vi "Demo_NOK_PART_COUNT.vi"(0 "Refnum in":T1, 1 "Station":string, 3 "Shift":i32, 5 "MAX BREAKDOWN ID":i32, 7 "Product code":string, 9 "TABLE NAME":string, 11 "error in (no error)":errorcluster, 12 "REJECTION COUNT":i32) -> (4 "Refnum out":T1, 6 "REJ COUNT":i32, 15 "error out":errorcluster)   [LabVIEW 2017]
uses:
  <vilib>/addons/database/Connection.llb/Conn ObjectReference.ctl
  <vilib>/addons/database/NI_Database_API.lvlib
  <userlib>/_OpenG.lib/comparison/comparison.llb/I32 Changed__ogtk.vi
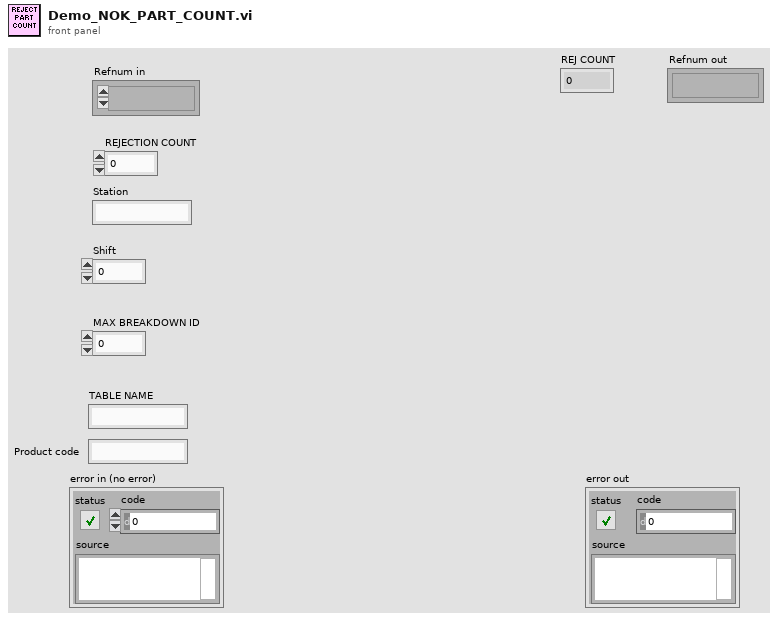
[diagram p1: front panel]
types:
  T1 = typedef "NI_Database_API.lvlib/Conn ObjectReference.ctl" = refnum<k1>
  T2 = typedef "LVDateTimeRec.ctl" = cluster{"fractional second":dbl, "second":i32, "minute":i32, "hour":i32, "day of month":i32, "month":i32, "year":i32, "day of week":i32, "day of year":i32, "DST":i32}
  T3 = cluster{i32, "Station":string, i32, "Shift":i32, "date/time string":string, "Date String":string, "Product code":string}
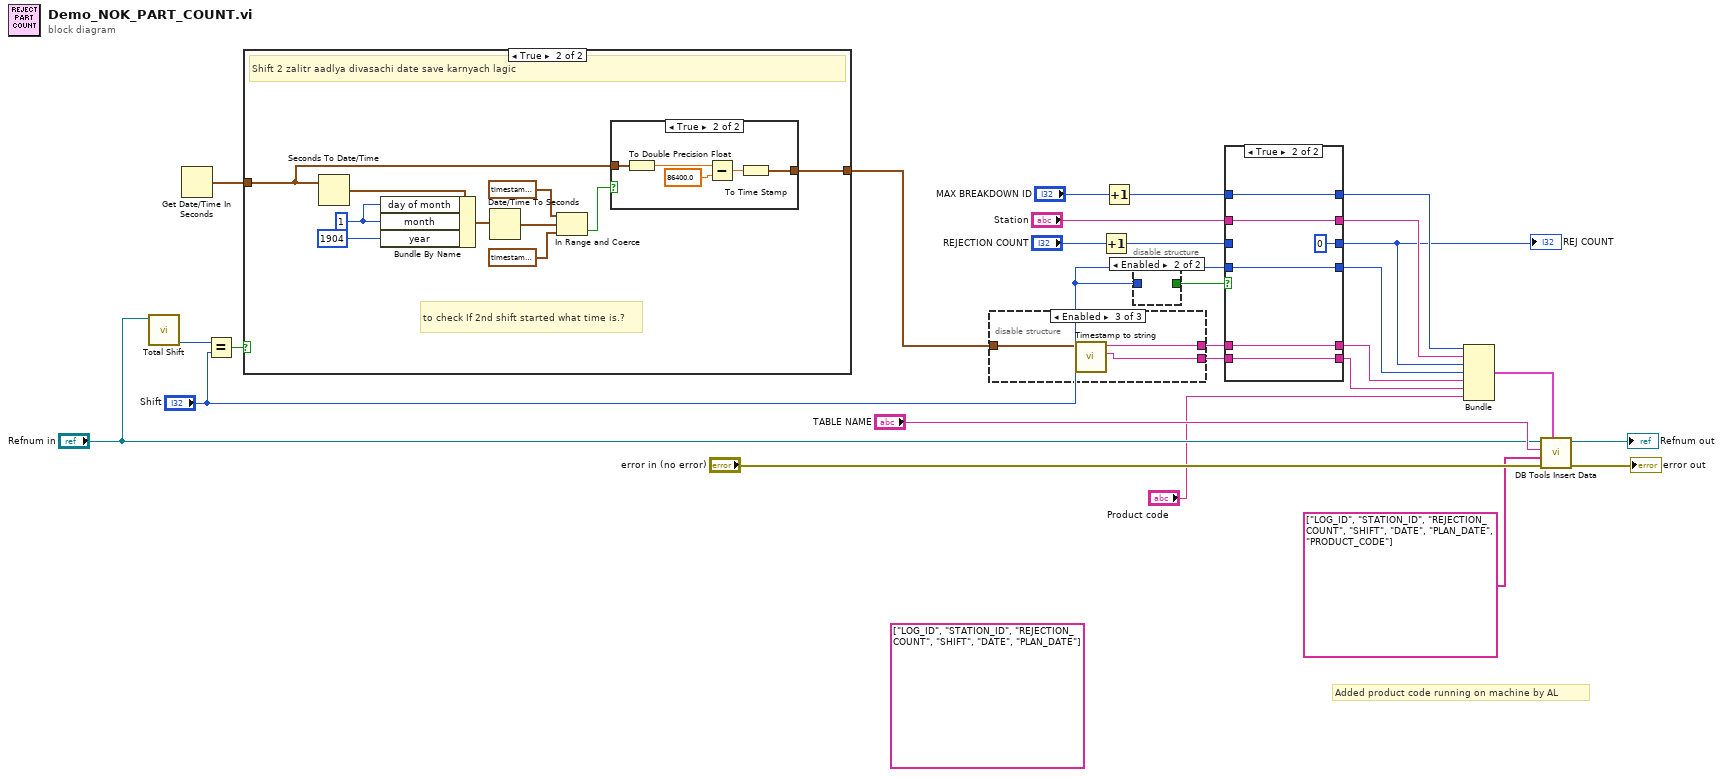
[diagram p0: block diagram]
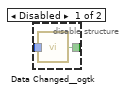
[diagram p2: hidden frame]
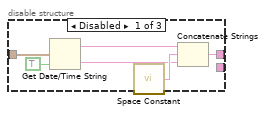
[diagram p3: hidden frame]
diagram:
  (unwired) string[] ["LOG_ID", "STATION_ID", "REJECTION_COUNT", "SHIFT", "DATE", "PLAN_DATE"] ("columns")
  # "Added product code running on machine by AL"
  n1 = call "Total Shift.vi"("connection reference"="Refnum in") -> ("Total Shifts"=w10:i32)  [unwired: 9 in, 1 out]
  n2 = Get Date/Time In Seconds() -> (seconds since 1Jan1904=w9:timestamp)
  n3 = Equal?(x=w10, y="Shift") -> (x = y?=w11:bool)
  n4 = case shown="True" w11 {
    tunnel: w9 -> [w28 w29]
    tunnel: [w28 w30] -> w8
    frame False {
    }
    frame True {
      w35 = 1 ("day of month")
      # "to check If 2nd shift started what time is.?"
      # "Shift 2 zalitr aadlya divasachi date save karnyach lagic"
      n5 = Seconds To Date/Time(time stamp (now)=w29) -> (date time rec=w36:T2)  [unwired: 1 in]
      n6 = Bundle By Name(cluster=w36, "day of month"=w35, "month"=w35, "year"=1904) -> (w38:T2)
      n7 = Date/Time To Seconds(2:w38) -> (0:w34:timestamp)  [unwired: 1 in]
      n8 = In Range and Coerce(upper limit=timestamp(5399 s since 1904-01-01), x=w34, lower limit=timestamp(-19800 s since 1904-01-01)) -> (In Range?=w31:bool)  [unwired: 1 out]
      n9 = case shown="True" w31 {
        tunnel: [w39 w41] -> w30
        tunnel: w29 -> [w39 w40]
        frame False {
        }
        frame True {
          n10 = To Double Precision Float(number=w40) -> (double precision float=w44:dbl)
          n11 = Subtract(x=w44, y=86400.0) -> (x-y=w42:dbl)
          n12 = To Time Stamp(1:w42) -> (0:w41:timestamp)
        }
      }
    }
  }
  n13 = disable-structure shown="Enabled" {
    disable-tunnel: w8 -> [w50 w51 w54]
    disable-tunnel: [w46 w51 w53] -> w5
    disable-tunnel: [_ _ w52] -> w4
    frame Disabled {
      n14 = Get Date/Time String(seconds (now)=w50, want seconds? (F)=TRUE) -> (date string=w47:string, time string=w48:string)  [unwired: 1 in]
      n15 = call <vilib>:"Space Constant.vi"() -> ("String"=w49:string)
      n16 = Concatenate Strings(w47, w49, w48) -> (w46:string)
    }
    frame Disabled {
    }
    frame Enabled {
      n17 = call "Timestamp to string.vi"("time stamp"=w54) -> ("Date String"=w52:string, "date/time string"=w53:string)  [unwired: 8 in, 1 out]
    }
  }
  n18 = Increment(x="REJECTION COUNT") -> (x+1=w15:i32)
  n19 = Increment(x="MAX BREAKDOWN ID") -> (x+1=w18:i32)
  n20 = disable-structure shown="Enabled" {
    disable-tunnel: [w56 _] -> w20
    disable-tunnel: "Shift" -> [w55 _]
    frame Disabled {
      n21 = call-poly <userlib>:"Data Changed__ogtk.vi"("I32"=w55) -> ("Changed"=w56:bool)
    }
    frame Enabled {
    }
  }
  n22 = case shown="True" w20 {
    tunnel: [w62 w68] -> w19
    tunnel: w18 -> [w62 w68]
    tunnel: [w61 w67] -> w17
    tunnel: "Station" -> [w61 w67]
    tunnel: [w60 0] -> w12
    tunnel: w15 -> [w60 _]
    tunnel: [w59 w66] -> w14
    tunnel: "Shift" -> [w59 w66]
    tunnel: [w58 w65] -> w13
    tunnel: w5 -> [w58 w65]
    tunnel: [w57 w63] -> w3
    tunnel: w4 -> [w57 w63]
    frame False {
    }
    frame True {
    }
  }
  "REJ COUNT" <- w12
  n23 = Bundle(w19, "Station"=w17, w12, "Shift"=w14, "date/time string"=w13, "Date String"=w3, "Product code"="Product code") -> (w25:T3)  [unwired: 1 in]
  n24 = call <vilib>:"DB Tools Insert Data.vi"("data"=w25, "error in (no error)"="error in (no error)", "columns"=string[] ["LOG_ID", "STATION_ID", "REJECTION_COUNT", "SHIFT", "DATE", "PLAN_DATE", "PRODUCT_CODE"], "table"="TABLE NAME", "connection reference"="Refnum in") -> ("error out"=→"error out":errorcluster, "connection reference out"=→"Refnum out":T1)  [unwired: 5 in]
